vi "Get Messages.vi"(0 "Web App Handle In":T2, 1 "Items/Page":u16(ring)=10 items=["100"=100, "50"=50, "20"=20, "10"=10, "5"=5, "1"=1], 2 "Page #":i32, 3 "error in":errorcluster) -> (7 "Web App Handle Out":T2, 8 "Message List":T1(array[cluster]), 10 "error out":errorcluster)   [LabVIEW 2013, in "Web Messaging API.lvlib"]
doc: "Reads a list of Messages from the Web Messaging service, more information can be found at https://myrio.niwsc.com"
uses:
  Web Messaging API.lvlib
  Web Messaging Handle.ctl
  <vilib>/Utility/error.llb/DialogType.ctl
  <vilib>/httpClient/LabVIEWHTTPClient.lvlib
panel:
  out "body":string
  in  "JSON Array":T1(array[cluster])
  out "headers":string
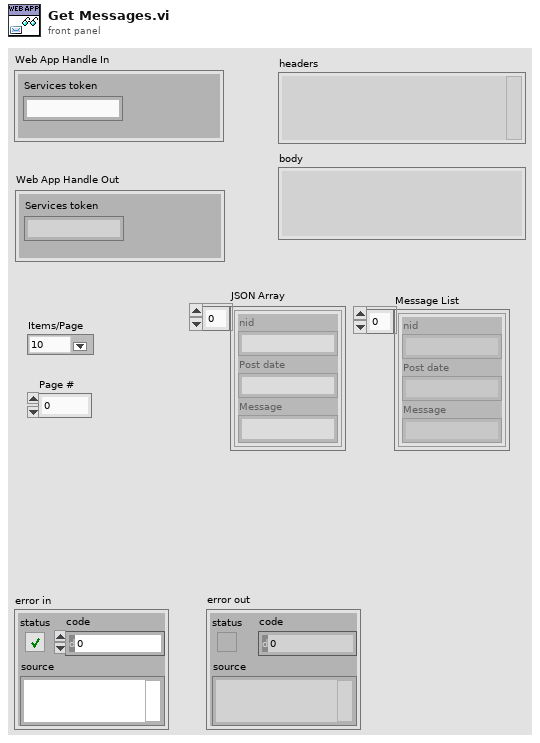
[diagram p1: front panel]
types:
  T1 = cluster{"nid":string, "Post date":string, "Message":string}[]
  T2 = typedef "Web Messaging API.lvlib/Web Messaging Handle.ctl" = cluster{"Services token":string}
  T3 = typedef "DialogType.ctl" = u16
  T4 = typedef "LabVIEWHTTPClient.lvlib/ClientHandle.ctl" = refnum<k1>
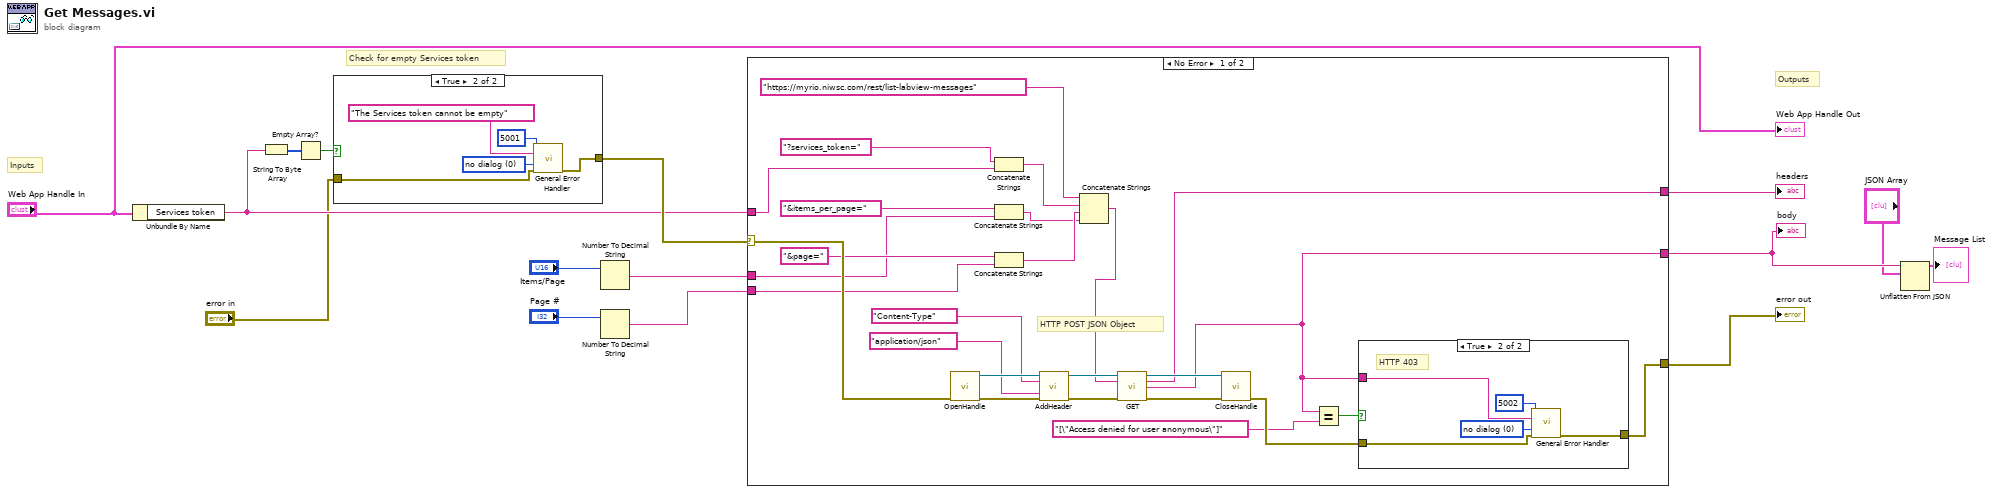
[diagram p0: block diagram]
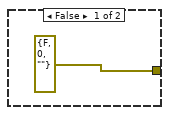
[diagram p2: hidden frame]
diagram:
  # "Check for empty Services token"
  # "Outputs"
  # "Inputs"
  n1 = Unbundle By Name("Web App Handle In") -> ("Services token"=w10:string)
  n2 = String To Byte Array(string=w10) -> (unsigned byte array=w13:u8[])
  n3 = Empty Array?(array=w13) -> (empty?=w12:bool)
  n4 = case shown="True" w12 {
    tunnel: [w16 w19] -> w11
    tunnel: "error in" -> [w16 w17]
    frame False {
    }
    frame True {
      w20 = T3 0 items=["no dialog", "OK message", "continue or stop message", "OK message + warnings", "continue/stop + warnings"] ("type of dialog (OK msg:1)")
      n5 = call <vilib>:"General Error Handler.vi"("[error code] (0)"=5001, "[error source] (\" \")"="The Services token cannot be empty" ("[error source] (\" \")"), "type of dialog (OK msg:1)"=w20, "error in (no error)"=w17) -> ("error out"=w19:errorcluster)  [unwired: 7 in, 4 out]
    }
  }
  n6 = Number To Decimal String(number="Items/Page") -> (decimal integer string=w4:string)  [unwired: 1 in]
  n7 = Number To Decimal String(number="Page #") -> (decimal integer string=w2:string)  [unwired: 1 in]
  n8 = case shown="No Error" w11 {
    selector: w11 -> [w43 w54]
    tunnel: w10 -> [w26 _]
    tunnel: [w36 _] -> w15
    tunnel: [w35 _] -> w8
    tunnel: [w41 w54] -> w14
    tunnel: w4 -> [w25 _]
    tunnel: w2 -> [w24 _]
    frame No Error {
      # "HTTP POST JSON Object"
      n9 = call <vilib>:"OpenHandle.vi"("error in (no error)"=w43) -> ("client handle out"=w47:T4, "error out"=w46:errorcluster)  [unwired: 13 in]
      n10 = Concatenate Strings("?services_token=" ("value"), w26) -> (w31:string)
      n11 = Concatenate Strings("&items_per_page=" ("string"), w25) -> (w22:string)
      n12 = Concatenate Strings("&page=" ("string"), w24) -> (w23:string)
      n13 = call <vilib>:"AddHeader.vi"("client handle"=w47, "header"="Content-Type", "value"="application/json", "error in (no error)"=w46) -> ("client handle out"=w34:T4, "error out"=w33:errorcluster)  [unwired: 10 in]
      n14 = Concatenate Strings("https://myrio.niwsc.com/rest/list-labview-messages" ("value"), w31, w23, w22) -> (w27:string)
      n15 = call <vilib>:"GET.vi"("client handle"=w34, "url"=w27, "error in (no error)"=w33) -> ("client handle out"=w37:T4, "headers"=w36:string, "body"=w35:string, "error out"=w38:errorcluster)  [unwired: 9 in]
      n16 = call <vilib>:"CloseHandle.vi"("client handle"=w37, "error in (no error)"=w38) -> ("error out"=w42:errorcluster)  [unwired: 13 in]
      n17 = Equal?(x=w35, y="[\"Access denied for user anonymous\"]") -> (x = y?=w39:bool)
      n18 = case shown="True" w39 {
        tunnel: [errorcluster {"status"=FALSE, "code"=0, "source"=""} ("error out") w52] -> w41
        tunnel: w42 -> [_ w50]
        tunnel: w35 -> [_ w49]
        frame False {
        }
        frame True {
          w53 = T3 0 items=["no dialog", "OK message", "continue or stop message", "OK message + warnings", "continue/stop + warnings"] ("type of dialog (OK msg:1)")
          # "HTTP 403"
          n19 = call <vilib>:"General Error Handler.vi"("[error code] (0)"=5002, "[error source] (\" \")"=w49, "type of dialog (OK msg:1)"=w53, "error in (no error)"=w50) -> ("error out"=w52:errorcluster)  [unwired: 7 in, 4 out]
        }
      }
    }
    frame Error {
    }
  }
  "headers" <- w15
  "error out" <- w14
  "body" <- w8
  n20 = Unflatten From JSON(JSON string=w8, type and defaults="JSON Array") -> (value=→"Message List":T1)  [unwired: 5 in, 1 out]
  "Web App Handle Out" <- "Web App Handle In"
